vi "Check Star.vi"(7 "Packed refs":T1, 8 "error in (no error)":errorcluster, 11 "Board Game in":refnum<class "Board Game.lvclass">) -> (0 "error out":errorcluster, 3 "Board Game out":refnum<class "Board Game.lvclass">)   [LabVIEW 2021, in "Board Game.lvclass"]
uses:
  Board Game.lvclass
  Application/Packed Refs.ctl
  GameEl_class/private/Enum Direction.ctl
  Board Game.lvclass/Board Game.ctl
  GameEl_class/GameEl.lvclass/GameEl.ctl
  Snake_class/Snake.lvclass/Snake.ctl
  Star/Star.lvclass/Star.ctl
  Imposible_Snake_v2/LVApp/Modules/Sound Manager/Typedefs/Sound Effects.ctl
  <vilib>/numeric/Random Number (Range) U64.vi
  GameEl_class/Write Visible.vi
  Snake_class/Write Star.vi
  Star/Write Eat time.vi
  Star/Read STAR.vi
  GameEl_class/Read Visible.vi
  GameEl_class/Read position.vi
  Star/Read Eat time.vi
  Star/Read Init Star.vi
  Snake_class/Read Snake Head.vi
  Snake_class/Read Star.vi
  <vilib>/numeric/sub_Random U32.vi
  Star/Star.lvclass
  C:/Users/poche/Programs/LabVIEW/imposible snake/GameEl_class/GameEl.lvclass
  Snake_class/Snake.lvclass
  Shield/Shield.lvclass
  GameEl_class/GameEl.lvclass
  Imposible_Snake_v2/LVApp/Modules/Sound Manager/Sound Manager.lvlib
  Application/Game.lvclass
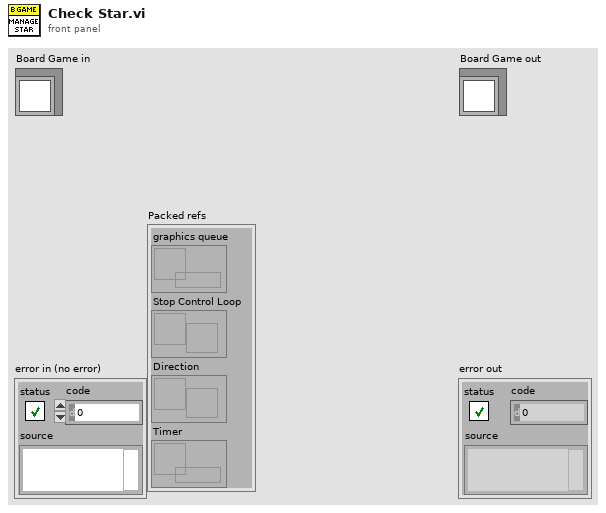
[diagram p1: front panel]
types:
  T1 = typedef "Game.lvclass/Packed Refs.ctl" = cluster{"graphics queue":refnum<queue>, "Stop Control Loop":refnum<user-event>, "Direction":refnum<notifier>, "Timer":refnum<data-value>}
  T2 = typedef "Sound Manager.lvlib/Sound Effects.ctl" = enum16{"Bomb In", "Bomb Out", "Bomb Touched", "Game Over", "Victory", "Eat", "10 Fruits", "Eat2", "Eat3", "Eat4", "MaxShield", "Shield", "10p", "Grape In", "Grape Out", "20p", "30p", "40p", "50p", "60p", "70p", "80p", "90p", "100p", "All shields cracked", "Mouse In", "Mouse Out", "Mouse Eaten", "Grape Eaten", "States Recover", "Broken Shield", "Bonus", "Happy Time", "explode", "Game over musica", "Back Music", "Shield Catch", "Evil lough", "Cricket In", "Cricket eaten", "Lets Go", "Jump1", "Jump2", "Jump3", "Unstoppable", "Troll Music", "winner", "menu"}
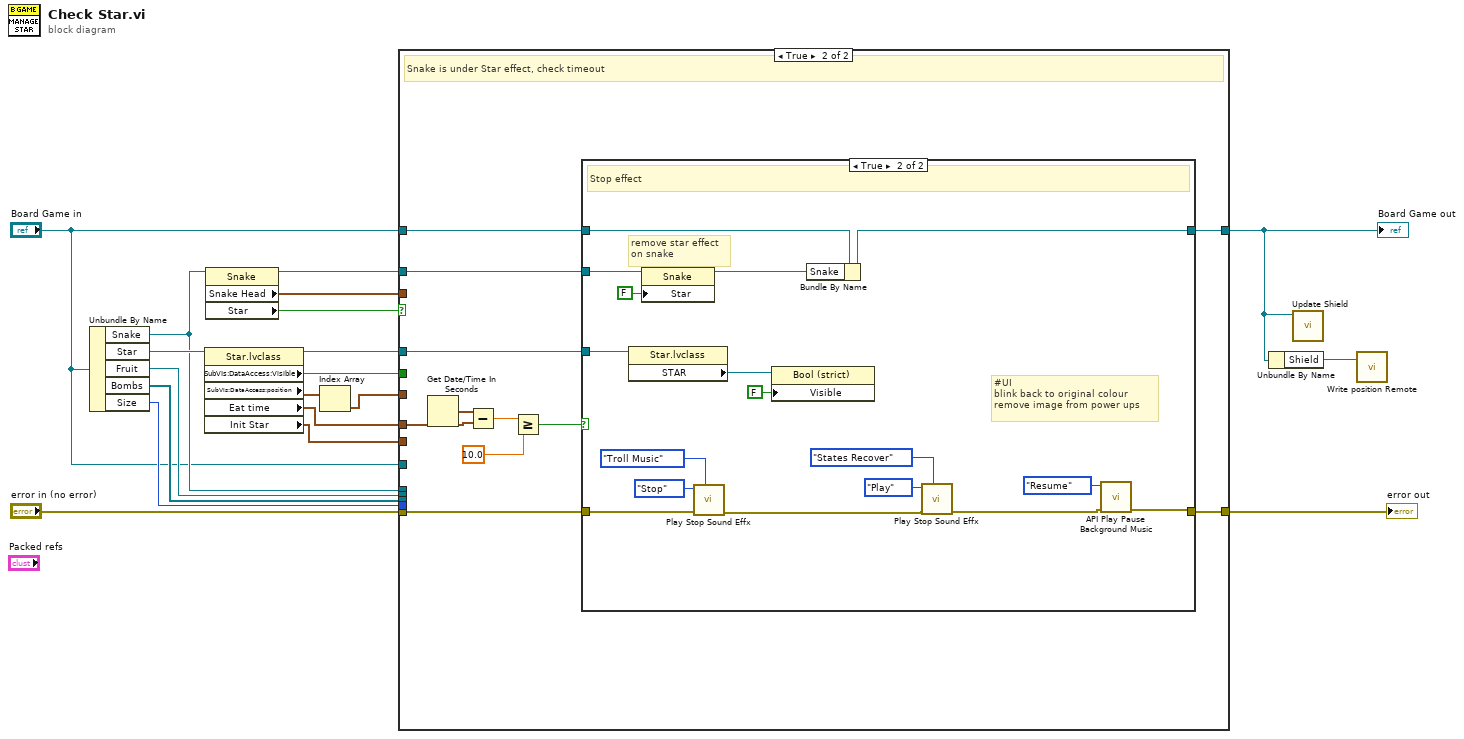
[diagram p0: block diagram]
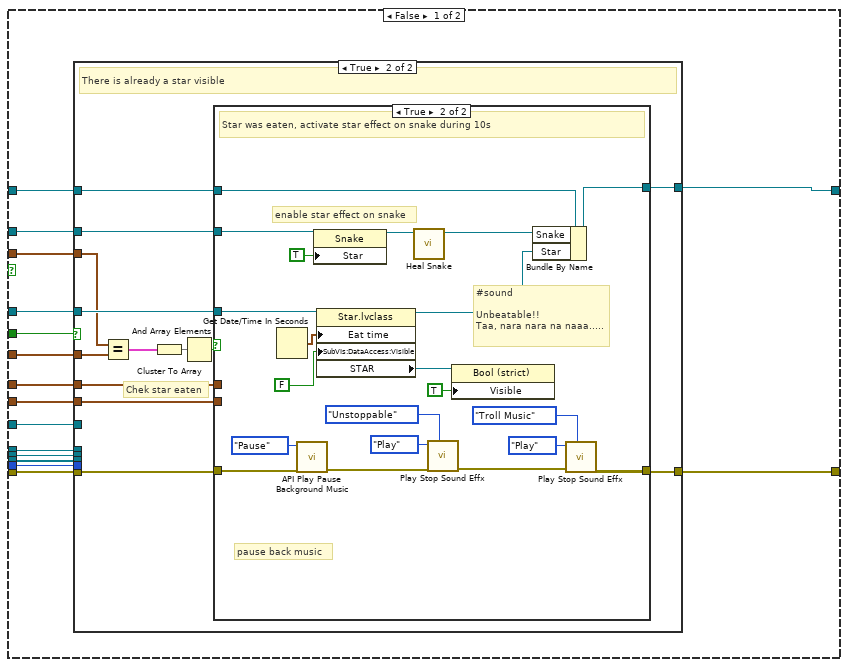
[diagram p2: hidden frame]
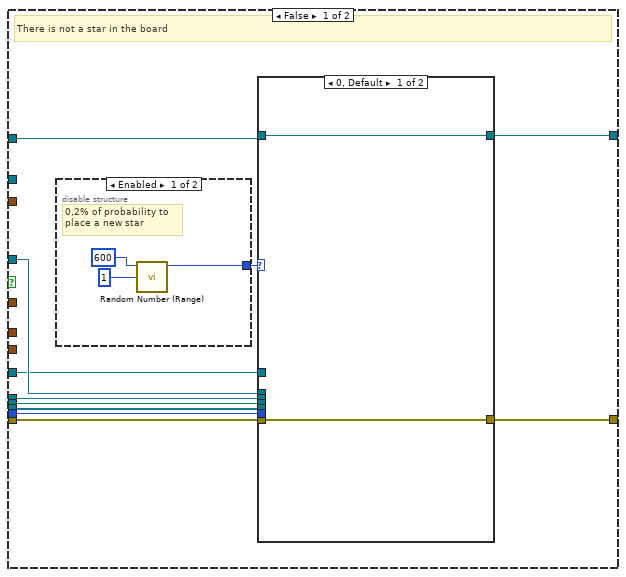
[diagram p3: hidden frame]
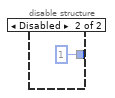
[diagram p4: hidden frame]
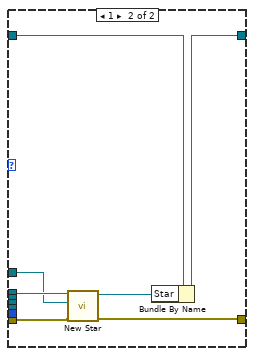
[diagram p5: hidden frame]
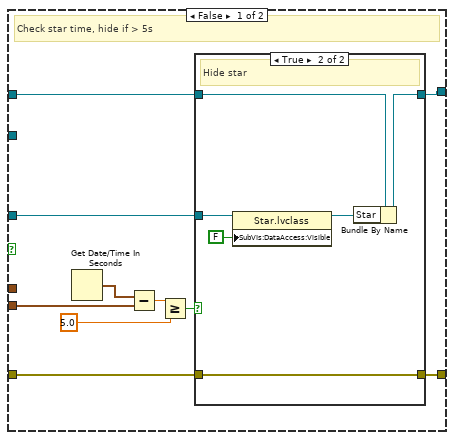
[diagram p6: hidden frame]
diagram:
  n1 = Unbundle By Name("Board Game in") -> ("Snake"=w12:refnum<class "Snake.lvclass">, "Star"=w19:refnum<class "Star.lvclass">, "Fruit"=w11:refnum<class "Fruit.lvclass">, "Bombs"=w10:refnum<class "Bomb.lvclass">[], "Size"=w9:u16)
  n2 = property class="Star.lvclass"(reference=w19) -> (reference out=w15:refnum<class "Star.lvclass">, "SubVIs:DataAccess:Visible"=w16:bool, "SubVIs:DataAccess:position"=w14:cluster{"x":dbl, "y":dbl}[], "Eat time"=w3:timestamp, "Init Star"=w2:timestamp)  [unwired: 1 in, 1 out]
  n3 = property class="Snake"(reference=w12) -> (reference out=w5:refnum<class "Snake.lvclass">, "Snake Head"=w13:cluster{"x":dbl, "y":dbl}, "Star"=w4:bool)  [unwired: 1 in, 1 out]
  n4 = Index Array(array=w14) -> (element=w8:cluster{"x":dbl, "y":dbl})  [unwired: 1 in]
  n5 = case shown="True" w4 {
    tunnel: "error in (no error)" -> [w35 w118]
    tunnel: [w34 w115] -> w17
    tunnel: "Board Game in" -> [w33 w117]
    tunnel: w16 -> [w32 _]
    tunnel: w15 -> [w31 w112]
    tunnel: w13 -> [w30 _]
    tunnel: w12 -> [w29 _]
    tunnel: w11 -> [w28 _]
    tunnel: w10 -> [w27 _]
    tunnel: w9 -> [w26 _]
    tunnel: w8 -> [w25 _]
    tunnel: [w24 w116] -> w7
    tunnel: w5 -> [w23 w113]
    tunnel: w3 -> [w22 w121]
    tunnel: w2 -> [w21 _]
    tunnel: "Board Game in" -> [w20 _]
    frame False {
      n6 = case shown="True" w32 {
        tunnel: w35 -> [w46 w67]
        tunnel: [w45 w66] -> w34
        tunnel: w33 -> [w44 w65]
        tunnel: [w43 w64] -> w24
        tunnel: w31 -> [w42 w72]
        tunnel: w25 -> [_ w71]
        tunnel: w30 -> [_ w70]
        tunnel: w29 -> [w41 _]
        tunnel: w28 -> [w40 _]
        tunnel: w27 -> [w39 _]
        tunnel: w26 -> [w38 _]
        tunnel: w23 -> [_ w62]
        tunnel: w22 -> [_ w61]
        tunnel: w21 -> [_ w60]
        tunnel: w20 -> [w37 _]
        frame False {
          # "There is not a star in the board"
          n7 = disable-structure shown="Enabled" {
            disable-tunnel: [w47 u64 1 ("number")] -> w36
            frame Enabled {
              # "0,2% of probability to \nplace a new star"
              n8 = call-poly <vilib>:"Random Number (Range).vi"("lower bound (0)"=u64 1, "upper bound (100)"=u64 600) -> ("number"=w47:u64)  [unwired: 9 in]
            }
            frame Disabled {
            }
          }
          n9 = case shown="0, Default" w36 {
            tunnel: w46 -> [w51 w56]
            tunnel: [w51 w55] -> w45
            tunnel: w44 -> [w52 w59]
            tunnel: [w52 w58] -> w43
            tunnel: w42 -> [_ w57]
            tunnel: w41 -> [_ _]
            tunnel: w40 -> [_ _]
            tunnel: w39 -> [_ _]
            tunnel: w38 -> [_ _]
            tunnel: w37 -> [_ w53]
            frame 0, Default {
            }
            frame 1 {
              n10 = call "New Star.vi"("error in (no error)"=w56, "Board Game in"=w53, "Star in"=w57) -> ("error out"=w55:errorcluster, "Star out"=w54:refnum<class "Star.lvclass">)  [unwired: 7 in]
              n11 = Bundle By Name(cluster=w59, "Star"=w54) -> (w58:refnum<class "Board Game.lvclass">)
            }
          }
        }
        frame True {
          # "Chek star eaten"
          # "There is already a star visible"
          n12 = Equal?(x=w70, y=w71) -> (x = y?=w68:cluster{"x":bool, "y":bool})
          n13 = Cluster To Array(cluster=w68) -> (array=w69:bool[])
          n14 = And Array Elements(Boolean array=w69) -> (logical AND=w63:bool)
          n15 = case shown="True" w63 {
            tunnel: w72 -> [w74 w107]
            tunnel: w67 -> [w77 w92]
            tunnel: [w76 w95] -> w66
            tunnel: w65 -> [w78 w111]
            tunnel: [w75 w110] -> w64
            tunnel: w62 -> [_ w109]
            tunnel: w61 -> [_ _]
            tunnel: w60 -> [w73 _]
            frame False {
              # "Check star time, hide if > 5s"
              n16 = Get Date/Time In Seconds() -> (seconds since 1Jan1904=w82:timestamp)
              n17 = Subtract(x=w82, y=w73) -> (x-y=w81:dbl)
              n18 = Greater Or Equal?(x=w81, y=5.0) -> (x >= y?=w79:bool)
              n19 = case shown="True" w79 {
                tunnel: w78 -> [w84 w89]
                tunnel: w77 -> [w83 w90]
                tunnel: [w83 w90] -> w76
                tunnel: [w84 w88] -> w75
                tunnel: w74 -> [_ w87]
                frame False {
                }
                frame True {
                  # "Hide star"
                  n20 = property class="Star.lvclass"(reference=w87, "SubVIs:DataAccess:Visible"=FALSE ("Visible")) -> (reference out=w86:refnum<class "Star.lvclass">)  [unwired: 1 in, 1 out]
                  n21 = Bundle By Name(cluster=w89, "Star"=w86) -> (w88:refnum<class "Board Game.lvclass">)
                }
              }
            }
            frame True {
              # "pause back music"
              # "#sound\n\nUnbeatable!!\nTaa, nara nara na naaa....."
              # "enable star effect on snake"
              # "Star was eaten, activate star effect on snake during 10s"
              n22 = Get Date/Time In Seconds() -> (seconds since 1Jan1904=w106:timestamp)
              n23 = call "API Play Pause Background Music.vi"("Error In"=w92, "Function"=enum16{"Pause", "Resume"}."Pause") -> ("error in (no error)"=w91:errorcluster)  [unwired: 9 in]
              n24 = property class="Snake"(reference=w109, "Star"=TRUE) -> (reference out=w108:refnum<class "Snake.lvclass">)  [unwired: 1 in, 1 out]
              n25 = property class="Star.lvclass"(reference=w107, "Eat time"=w106, "SubVIs:DataAccess:Visible"=FALSE ("Visible")) -> (reference out=w105:refnum<class "Star.lvclass">, "STAR"=w101:refnum<vi>)  [unwired: 1 in, 1 out]
              n26 = call "Heal Snake.vi"("Snake in"=w108) -> ("Snake out"=w104:refnum<class "Snake.lvclass">)  [unwired: 9 in, 1 out]
              n27 = call "Play Stop Sound Effx.vi"("Sound Effect"=Sound_Effects."Unstoppable", "Error In"=w91, "Function"=enum16{"Play", "Stop"}."Play") -> ("error in (no error)"=w94:errorcluster)  [unwired: 8 in]
              n28 = property class="Bool (strict)"(reference=w101, "Visible"=TRUE) -> ()  [unwired: 1 in, 2 out]
              n29 = Bundle By Name(cluster=w111, "Snake"=w104, "Star"=w105) -> (w110:refnum<class "Board Game.lvclass">)
              n30 = call "Play Stop Sound Effx.vi"("Sound Effect"=Sound_Effects."Troll Music", "Error In"=w94, "Function"=enum16{"Play", "Stop"}."Play") -> ("error in (no error)"=w95:errorcluster)  [unwired: 8 in]
            }
          }
        }
      }
    }
    frame True {
      # "Snake is under Star effect, check timeout"
      n31 = Get Date/Time In Seconds() -> (seconds since 1Jan1904=w122:timestamp)
      n32 = Subtract(x=w122, y=w121) -> (x-y=w120:dbl)
      n33 = Greater Or Equal?(x=w120, y=10.0) -> (x >= y?=w114:bool)
      n34 = case shown="True" w114 {
        tunnel: w118 -> [w123 w129]
        tunnel: w117 -> [w124 w141]
        tunnel: [w124 w140] -> w116
        tunnel: [w123 w126] -> w115
        tunnel: w113 -> [_ w139]
        tunnel: w112 -> [_ w136]
        frame False {
          # "Keep star effect"
        }
        frame True {
          # "remove star effect \non snake"
          # "#UI\nblink back to original colour\nremove image from power ups"
          # "Stop effect"
          n35 = property class="Star.lvclass"(reference=w136) -> ("STAR"=w135:refnum<vi>)  [unwired: 1 in, 2 out]
          n36 = property class="Snake"(reference=w139, "Star"=FALSE) -> (reference out=w137:refnum<class "Snake.lvclass">)  [unwired: 1 in, 1 out]
          n37 = call "Play Stop Sound Effx.vi"("Sound Effect"=Sound_Effects."Troll Music", "Error In"=w129, "Function"=enum16{"Play", "Stop"}."Stop") -> ("error in (no error)"=w128:errorcluster)  [unwired: 8 in]
          n38 = property class="Bool (strict)"(reference=w135, "Visible"=FALSE) -> ()  [unwired: 1 in, 2 out]
          n39 = Bundle By Name(cluster=w141, "Snake"=w137) -> (w140:refnum<class "Board Game.lvclass">)
          n40 = call "Play Stop Sound Effx.vi"("Sound Effect"=Sound_Effects."States Recover", "Error In"=w128, "Function"=enum16{"Play", "Stop"}."Play") -> ("error in (no error)"=w127:errorcluster)  [unwired: 8 in]
          n41 = call "API Play Pause Background Music.vi"("Error In"=w127, "Function"=enum16{"Pause", "Resume"}."Resume") -> ("error in (no error)"=w126:errorcluster)  [unwired: 9 in]
        }
      }
    }
  }
  "error out" <- w17
  "Board Game out" <- w7
  n42 = Unbundle By Name(w7) -> ("Shield"=w6:refnum<class "Shield.lvclass">)
  n43 = call "Update Shield.vi"("Board Game in"=w7) -> ()  [unwired: 11 in]
  n44 = call "Write position Remote.vi"("GameEl in"=w6) -> ()  [unwired: 10 in, 1 out]
